vi "DHTxx_Initial.vi"(8 "error in (no error)":errorcluster) -> (0 "error out":errorcluster, 3 "return type":i32)   [LabVIEW 2014, in "QwaveSys Raspberry Pi Library.lvlib"]
uses:
  QwaveSys Raspberry Pi Library.lvlib
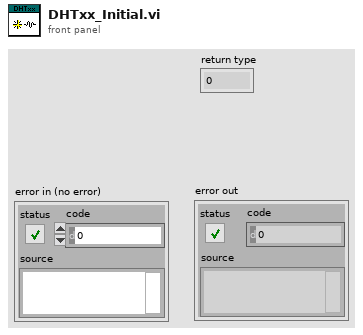
[diagram p1: front panel]
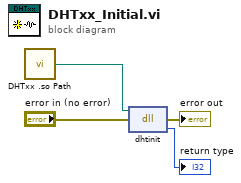
[diagram p0: block diagram]
diagram:
  n1 = call "DHTxx .so Path.vi"() -> ("DHTxx .so Path"=w1:path)  [unwired: 5 in]
  n2 = dll-call lib="libdht.so" fn="dhtinit"(path in=w1, error in="error in (no error)") -> (error out=→"error out":errorcluster, "return type"=→"return type":i32)  [unwired: 1 in, 1 out]
